vi "Write and Read Multiple Holding Registers.vi"(4 "read count":u16, 6 "read starting address":u16, 8 "error in (no error)":errorcluster, 9 "write values":u16[](array[numeric]), 10 "write starting address":u16, 11 "device data model in":refnum<class "Standard Data Model.lvclass">) -> (0 "error out":errorcluster, 1 "read values":u16[](array[numeric]), 3 "device data model out":refnum<class "Standard Data Model.lvclass">)   [LabVIEW 2018, in "SubVIs.lvlib" / "Standard Data Model.lvclass"]
doc: "Writes and reads the values of multiple register values in series. The <b>write values</b> are inserted starting at <b>write starting address</b> and the returned <b>read values</b> consists of <b>read count</b> holding registers starting at <b>read starting address</b>."
uses:
  Standard Data Model.lvclass
  Standard Data Model.lvclass/Standard Data Model.ctl
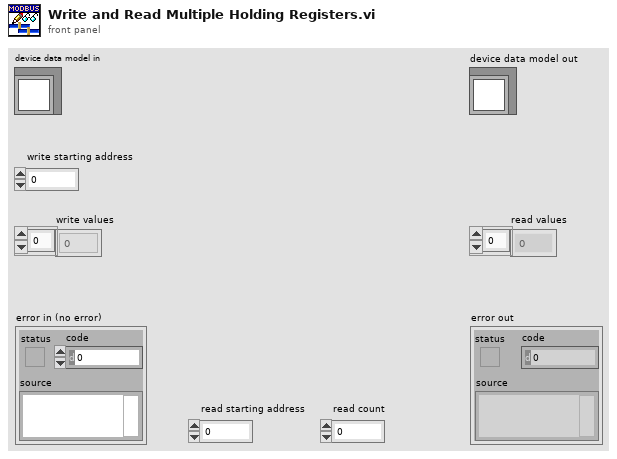
[diagram p1: front panel]
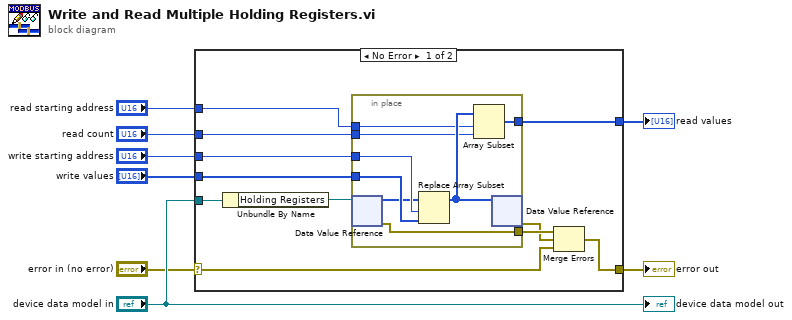
[diagram p0: block diagram]
diagram:
  n1 = case shown="No Error" "error in (no error)" {
    selector: "error in (no error)" -> [w10 w28]
    tunnel: [w19 w28] -> w8
    tunnel: "write values" -> [w17 _]
    tunnel: "write starting address" -> [w16 _]
    tunnel: [w15 _] -> w5
    tunnel: "read count" -> [w14 _]
    tunnel: "read starting address" -> [w13 _]
    tunnel: "device data model in" -> [w11 _]
    frame No Error {
      n2 = Unbundle By Name(w11) -> ("Holding Registers"=w18:refnum<data-value>)
      n3 = in-place {
        in-place-border: w17 -> [w27]
        in-place-border: w16 -> [w26]
        in-place-border: [w23] -> w15
        in-place-border: w14 -> [w20]
        in-place-border: w13 -> [w22]
        in-place-border: [w21] -> w12
        n4 = in-place-dvr #1(w18) -> (w25:u16[], w21:errorcluster)
        n5 = Replace Array Subset(array=w25, new element=w27, index=w26) -> (w24:u16[])
        n6 = Array Subset(array=w24, index=w22, length=w20) -> (w23:u16[])
        n7 = in-place-dvr #1(w24) -> (w9:errorcluster)  [unwired: 1 out]
      }
      n8 = Merge Errors(w12, w9, w10) -> (w19:errorcluster)
    }
    frame Error {
    }
  }
  "error out" <- w8
  "read values" <- w5
  "device data model out" <- "device data model in"
